vi "DCPower Specific Logic.vi"(0 "instrument handle":refnum<k15>, 5 "session":T1, 9 "Measurement Configuration":T4={"pin_names"=[], "voltage_level"=6.0, "voltage_level_range"=6.0, "current_limit"=0.01, "current_limit_range"=0.01, "source_delay"=0.0}, 11 "error in":errorcluster) -> (3 "Sites":i32[](array[numeric]), 4 "instrument handle out":refnum<k15>, 6 "Voltage measurements":dbl[](array[numeric]), 8 "Current measurements":dbl[](array[numeric]), 10 "In Compliance":bool[](array[boolean]), 14 "Pin or relay names":string[](array[string]), 15 "error out":errorcluster)   [LabVIEW 2020, in "NIDCPowerSourceDCVoltage.lvlib"]
uses:
  NIDCPowerSourceDCVoltage.lvlib
  Measurement Configuration.ctl
  <vilib>/MeasurementLink/MeasurementLink Session Management Client/RPC Messages/ni_measurementlink_sessionmanagement_v1_SessionInformation.ctl
  <vilib>/MeasurementLink/MeasurementLink Session Management Client/RPC Messages/nidevice_grpc_Session.ctl
  <vilib>/MeasurementLink/MeasurementLink Session Management Client/RPC Messages/ni_measurementlink_sessionmanagement_v1_ChannelMapping.ctl
  <instrlib>/niDCPower/nidcpower.llb/niDCPower Source Mode.ctl
  <instrlib>/niDCPower/nidcpower.llb/niDCPower Output Function.ctl
  <instrlib>/niDCPower/nidcpower.llb/niDCPower Wait For Event - Event.ctl
  <vilib>/MeasurementLink/MeasurementLink Session Management Client/MeasurementLink Session Management Client.lvlib
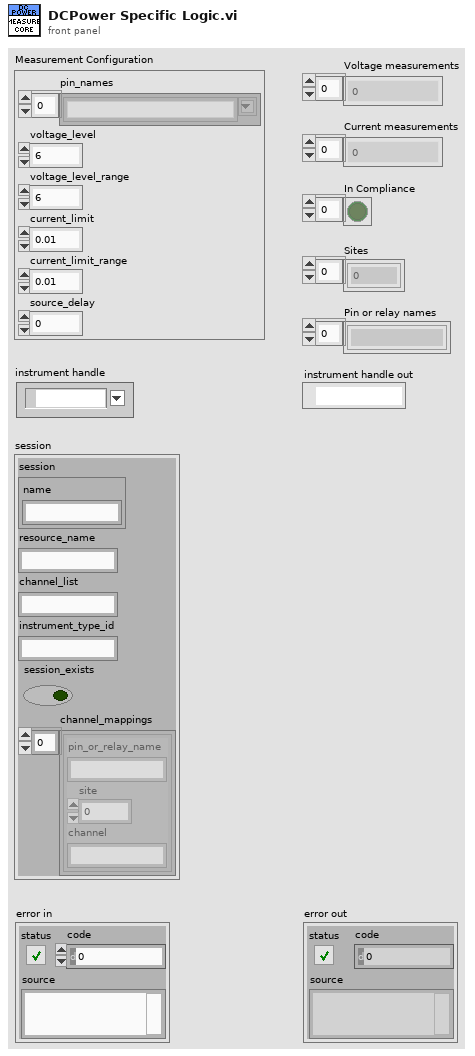
[diagram p1: front panel]
types:
  T1 = typedef "MeasurementLink Session Management Client.lvlib/ni_measurementlink_sessionmanagement_v1_SessionInformation.ctl" = cluster{"session":T2, "resource_name":string, "channel_list":string, "instrument_type_id":string, "session_exists":bool, "channel_mappings":T3[]}
  T2 = typedef "MeasurementLink Session Management Client.lvlib/nidevice_grpc_Session.ctl" = cluster{"name":string}
  T3 = typedef "MeasurementLink Session Management Client.lvlib/ni_measurementlink_sessionmanagement_v1_ChannelMapping.ctl" = cluster{"pin_or_relay_name":string, "site":i32, "channel":string}
  T4 = typedef "NIDCPowerSourceDCVoltage.lvlib/Measurement Configuration.ctl" = cluster{"pin_names":string[], "voltage_level":dbl, "voltage_level_range":dbl, "current_limit":dbl, "current_limit_range":dbl, "source_delay":dbl}
  T5 = typedef "niDCPower Wait For Event - Event.ctl" = i32
  T6 = typedef "niDCPower Output Function.ctl" = i32
  T7 = typedef "niDCPower Source Mode.ctl" = i32
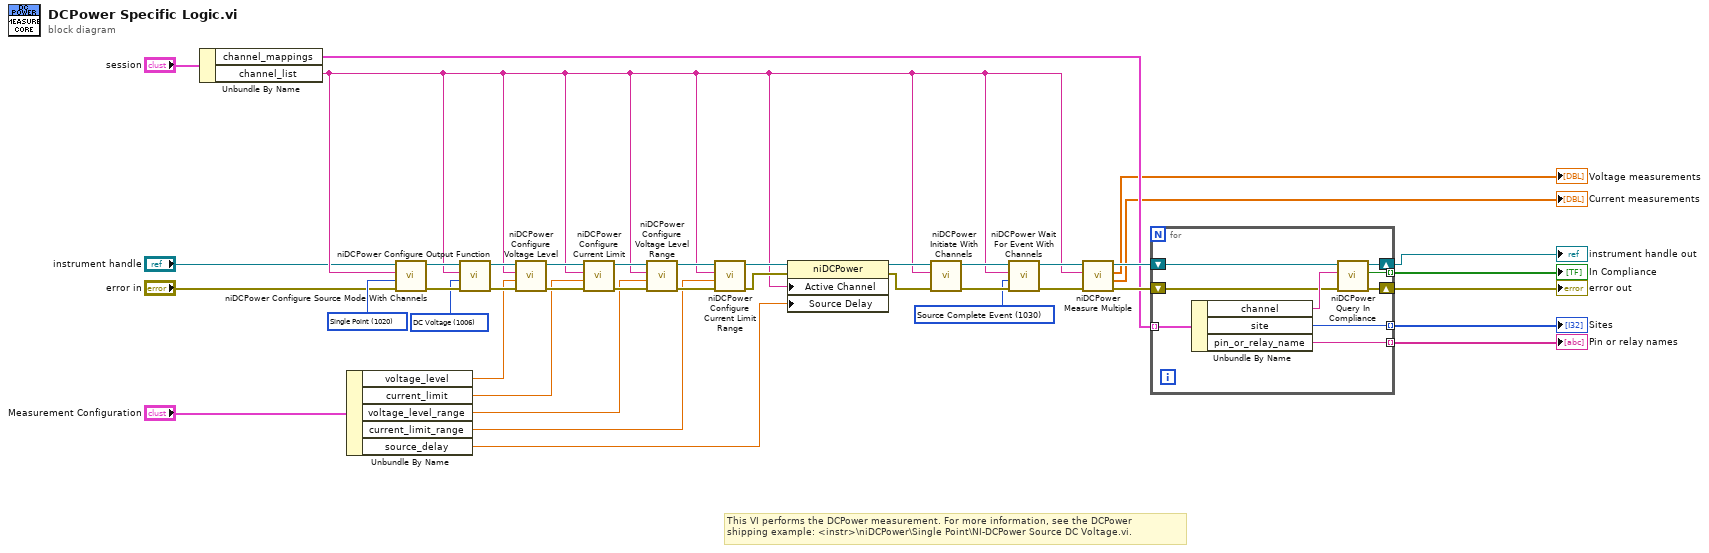
[diagram p0: block diagram]
diagram:
  w19 = T5 1030 items=["Source Complete Event"=1030, "Measure Complete Event"=1031, "Sequence Iteration Complete Event"=1032, "Sequence Engine Done Event"=1033, "Pulse Complete Event"=1051, "Ready For Pulse Trigger Event"=1052] ("event")
  w22 = T6 1006 items=["DC Voltage"=1006, "DC Current"=1007, "Pulse Voltage"=1049, "Pulse Current"=1050] ("output function")
  w23 = T7 1020 items=["Single Point"=1020, "Sequence"=1021] ("source mode")
  # "This VI performs the DCPower measurement. For more information, see the DCPower\nshipping example: <instr>\\niDCPower\\Single Point\\NI-DCPower Source DC Voltage.vi."
  n1 = Unbundle By Name("session") -> ("channel_mappings"=w11:T3[], "channel_list"=w14:string)
  n2 = Unbundle By Name("Measurement Configuration") -> ("voltage_level"=w21:dbl, "current_limit"=w20:dbl, "voltage_level_range"=w17:dbl, "current_limit_range"=w16:dbl, "source_delay"=w15:dbl)
  n3 = call <instrlib>:"niDCPower Configure Source Mode With Channels.vi"("error in (no error)"="error in", "source mode"=w23, "channel name"=w14, "instrument handle"="instrument handle") -> ("error out"=w39:errorcluster, "instrument handle out"=w38:refnum<k15>)  [unwired: 6 in]
  n4 = call <instrlib>:"niDCPower Configure Output Function.vi"("error in (no error)"=w39, "output function"=w22, "channel name"=w14, "instrument handle"=w38) -> ("error out"=w24:errorcluster, "instrument handle out"=w25:refnum<k15>)  [unwired: 6 out]
  n5 = call <instrlib>:"niDCPower Configure Voltage Level.vi"("error in (no error)"=w24, "voltage level"=w21, "channel name"=w14, "instrument handle"=w25) -> ("error out"=w40:errorcluster, "instrument handle out"=w41:refnum<k15>)  [unwired: 6 out]
  n6 = call <instrlib>:"niDCPower Configure Current Limit.vi"("error in (no error)"=w40, "current limit"=w20, "channel name"=w14, "instrument handle"=w41) -> ("error out"=w37:errorcluster, "instrument handle out"=w36:refnum<k15>)  [unwired: 1 in, 5 out]
  n7 = call <instrlib>:"niDCPower Configure Voltage Level Range.vi"("error in (no error)"=w37, "voltage level range"=w17, "channel name"=w14, "instrument handle"=w36) -> ("error out"=w35:errorcluster, "instrument handle out"=w34:refnum<k15>)  [unwired: 6 out]
  n8 = call <instrlib>:"niDCPower Configure Current Limit Range.vi"("error in (no error)"=w35, "current limit range"=w16, "channel name"=w14, "instrument handle"=w34) -> ("error out"=w30:errorcluster, "instrument handle out"=w33:refnum<k15>)  [unwired: 6 out]
  n9 = property class="niDCPower"(reference=w33, error in=w30, "Active Channel"=w14, "Source Delay"=w15) -> (reference out=w32:refnum<k15>, error out=w31:errorcluster)
  n10 = call <instrlib>:"niDCPower Initiate With Channels.vi"("error in (no error)"=w31, "channel name"=w14, "instrument handle"=w32) -> ("error out"=w27:errorcluster, "instrument handle out"=w29:refnum<k15>)  [unwired: 7 in]
  n11 = call <instrlib>:"niDCPower Wait For Event With Channels.vi"("error in (no error)"=w27, "event"=w19, "channel name"=w14, "instrument handle"=w29) -> ("error out"=w26:errorcluster, "instrument handle out"=w28:refnum<k15>)  [unwired: 6 in]
  n12 = call <instrlib>:"niDCPower Measure Multiple.vi"("error in (no error)"=w26, "channel name"=w14, "instrument handle"=w28) -> ("error out"=w12:errorcluster, "current measurements"=→"Current measurements":dbl[], "voltage measurements"=→"Voltage measurements":dbl[], "instrument handle out"=w13:refnum<k15>)  [unwired: 5 out]
  n13 = for {
    tunnel: w11 -> [w50] mode=indexing
    tunnel: [w49] -> w9 mode=indexing
    tunnel: [w48] -> w8 mode=indexing
    shift-right: [w45] -> w7
    shift-left: w13 -> [w46]
    shift-right: [w43] -> w4
    shift-left: w12 -> [w44]
    tunnel: [w42] -> w10 mode=indexing
    n14 = Unbundle By Name(w50) -> ("channel"=w47:string, "site"=w49:i32, "pin_or_relay_name"=w48:string)
    n15 = call <instrlib>:"niDCPower Query In Compliance.vi"("error in (no error)"=w44, "channel name"=w47, "instrument handle"=w46) -> ("error out"=w43:errorcluster, "in compliance?"=w42:bool, "instrument handle out"=w45:refnum<k15>)  [unwired: 6 out]
  }
  "error out" <- w4
  "instrument handle out" <- w7
  "In Compliance" <- w10
  "Sites" <- w9
  "Pin or relay names" <- w8
